vi "4461 - AI Read Data.vi"(8 "sampling info":cluster{"Fs":dbl, "#s":dbl}={"Fs"=1000.0, "#s"=1000.0} {"Fs" format="%.2p"}, 10 "AI Block Size":i32=5000, 11 "AI task":refnum<k21>[](array[refnum])=["", ""]) -> (1 "Backlog":u8(slide) scale=0.0..100.0, 2 "Input Signals":dbl[][](array[numeric]), 3 "Input Signals":waveform(dbl)[](array[waveform]))   [LabVIEW 2013]
uses:
  <vilib>/DAQmx/read.llb/DAQmx Read (Analog 2D DBL NChan NSamp).vi
  <resource>/objmgr/daqmx.rc
  <vilib>/DAQmx/read.llb/DAQmx Read (Analog 1D Wfm NChan NSamp).vi
panel:
  in  "AI Rate":dbl=10000.0 format="%.2f"
  in  "AI Buffer Size (s)":i32=10
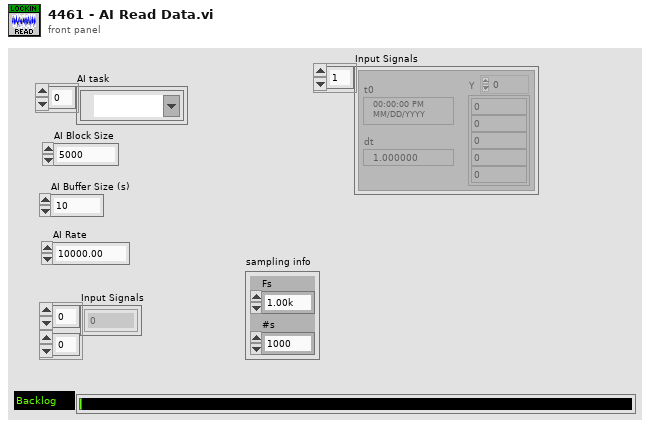
[diagram p1: front panel]
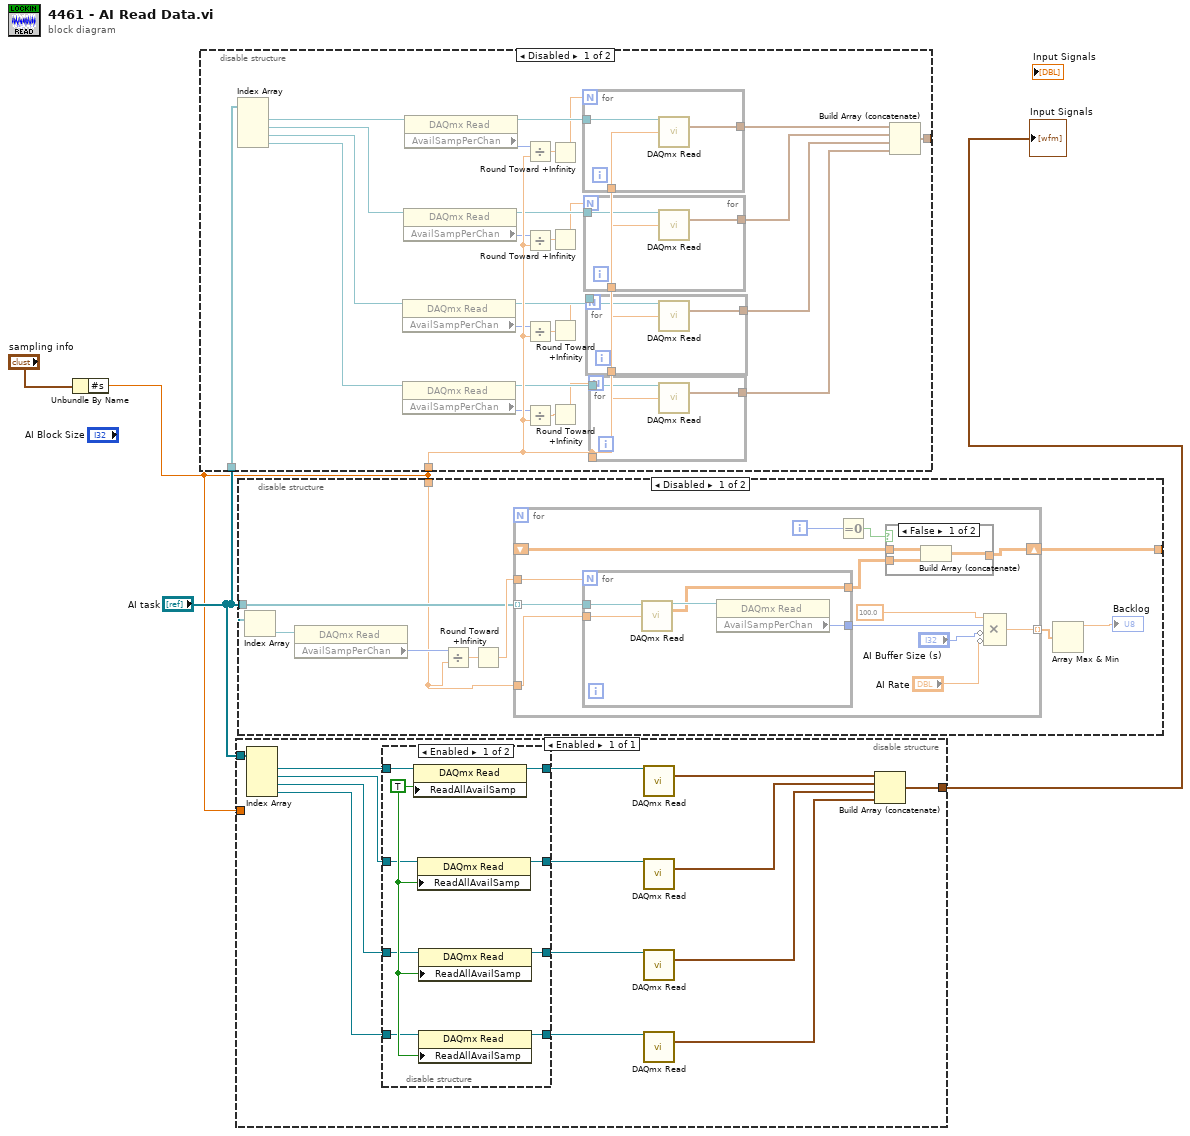
[diagram p0: block diagram]
diagram:
  n1 = Unbundle By Name("sampling info") -> ("#s"=w1:dbl)
  n2 = disable-structure shown="Disabled" {
    disable-tunnel: "AI task" -> [w31 _]
    disable-tunnel: w1 -> [w30 _]
    disable-tunnel: [w5 _] -> _
    frame Disabled {
      n3 = Index Array(array=w31) -> (element #1=w22:refnum<k21>, element #2=w23:refnum<k21>, element #3=w24:refnum<k21>, element #4=w25:refnum<k21>)  [unwired: 4 in]
      n4 = property class="DAQmx Read"(reference=w24) -> (reference out=w19:refnum<k21>, "AvailSampPerChan"=w15:u32)  [unwired: 1 in, 1 out]
      n5 = property class="DAQmx Read"(reference=w25) -> (reference out=w18:refnum<k21>, "AvailSampPerChan"=w16:u32)  [unwired: 1 in, 1 out]
      n6 = property class="DAQmx Read"(reference=w23) -> (reference out=w20:refnum<k21>, "AvailSampPerChan"=w14:u32)  [unwired: 1 in, 1 out]
      n7 = property class="DAQmx Read"(reference=w22) -> (reference out=w21:refnum<k21>, "AvailSampPerChan"=w17:u32)  [unwired: 1 in, 1 out]
      n8 = Divide(x=w17, y=w30) -> (x/y=w13:dbl)
      n9 = Divide(x=w14, y=w30) -> (x/y=w12:dbl)
      n10 = Divide(x=w15, y=w30) -> (x/y=w11:dbl)
      n11 = Divide(x=w16, y=w30) -> (x/y=w10:dbl)
      n12 = Round Toward +Infinity(x=w13) -> (ceil(x): smallest int >= x=w6:dbl)
      n13 = Round Toward +Infinity(x=w12) -> (ceil(x): smallest int >= x=w7:dbl)
      n14 = Round Toward +Infinity(x=w11) -> (ceil(x): smallest int >= x=w8:dbl)
      n15 = Round Toward +Infinity(x=w10) -> (ceil(x): smallest int >= x=w9:dbl)
      n16 = for {
        N: w6 -> [_]
        tunnel: [w43] -> w26
        tunnel: w21 -> [w42]
        tunnel: w30 -> [w41]
        n17 = call-poly <vilib>:"DAQmx Read.vi"("task/channels in"=w42, "number of samples per channel"=w41) -> ("data"=w43:waveform(dbl)[])  [unwired: 11 in, 2 out]
      }
      n18 = for {
        N: w7 -> [_]
        tunnel: [w40] -> w27
        tunnel: w20 -> [w39]
        tunnel: w30 -> [w38]
        n19 = call-poly <vilib>:"DAQmx Read.vi"("task/channels in"=w39, "number of samples per channel"=w38) -> ("data"=w40:waveform(dbl)[])  [unwired: 11 in, 2 out]
      }
      n20 = for {
        N: w8 -> [_]
        tunnel: [w37] -> w28
        tunnel: w19 -> [w36]
        tunnel: w30 -> [w35]
        n21 = call-poly <vilib>:"DAQmx Read.vi"("task/channels in"=w36, "number of samples per channel"=w35) -> ("data"=w37:waveform(dbl)[])  [unwired: 11 in, 2 out]
      }
      n22 = for {
        N: w9 -> [_]
        tunnel: [w34] -> w29
        tunnel: w18 -> [w33]
        tunnel: w30 -> [w32]
        n23 = call-poly <vilib>:"DAQmx Read.vi"("task/channels in"=w33, "number of samples per channel"=w32) -> ("data"=w34:waveform(dbl)[])  [unwired: 11 in, 2 out]
      }
      n24 = Build Array (concatenate)(w26, w27, w28, w29) -> (w5:waveform(dbl)[])
    }
    frame Enabled {
    }
  }
  n25 = disable-structure shown="Enabled" {
    disable-tunnel: "AI task" -> [w57]
    disable-tunnel: w1 -> [_]
    disable-tunnel: [w44] -> w4
    frame Enabled {
      n26 = Index Array(array=w57) -> (element #1=w56:refnum<k21>, element #2=w51:refnum<k21>, element #3=w50:refnum<k21>, element #4=w49:refnum<k21>)  [unwired: 4 in]
      n27 = disable-structure shown="Enabled" {
        disable-tunnel: w56 -> [w66 w70]
        disable-tunnel: [w65 w70] -> w55
        disable-tunnel: [w64 w67] -> w54
        disable-tunnel: [w63 w68] -> w53
        disable-tunnel: [w62 w69] -> w52
        disable-tunnel: w51 -> [w60 w69]
        disable-tunnel: w50 -> [w59 w68]
        disable-tunnel: w49 -> [w58 w67]
        frame Enabled {
          w61 = TRUE ("ReadAllAvailSamp")
          n28 = property class="DAQmx Read"(reference=w66, "ReadAllAvailSamp"=w61) -> (reference out=w65:refnum<k21>)  [unwired: 1 in, 1 out]
          n29 = property class="DAQmx Read"(reference=w60, "ReadAllAvailSamp"=w61) -> (reference out=w62:refnum<k21>)  [unwired: 1 in, 1 out]
          n30 = property class="DAQmx Read"(reference=w59, "ReadAllAvailSamp"=w61) -> (reference out=w63:refnum<k21>)  [unwired: 1 in, 1 out]
          n31 = property class="DAQmx Read"(reference=w58, "ReadAllAvailSamp"=w61) -> (reference out=w64:refnum<k21>)  [unwired: 1 in, 1 out]
        }
        frame Disabled {
        }
      }
      n32 = call-poly <vilib>:"DAQmx Read.vi"("task/channels in"=w55) -> ("data"=w48:waveform(dbl)[])  [unwired: 12 in, 2 out]
      n33 = call-poly <vilib>:"DAQmx Read.vi"("task/channels in"=w52) -> ("data"=w47:waveform(dbl)[])  [unwired: 12 in, 2 out]
      n34 = call-poly <vilib>:"DAQmx Read.vi"("task/channels in"=w53) -> ("data"=w46:waveform(dbl)[])  [unwired: 12 in, 2 out]
      n35 = call-poly <vilib>:"DAQmx Read.vi"("task/channels in"=w54) -> ("data"=w45:waveform(dbl)[])  [unwired: 12 in, 2 out]
      n36 = Build Array (concatenate)(w48, w47, w46, w45) -> (w44:waveform(dbl)[])
    }
  }
  "Input Signals" <- w4
  n37 = disable-structure shown="Disabled" {
    disable-tunnel: [w73 _] -> _
    disable-tunnel: "AI task" -> [w72 _]
    disable-tunnel: w1 -> [w71 _]
    frame Disabled {
      n38 = Index Array(array=w72) -> (element=w77:refnum<k21>)  [unwired: 1 in]
      n39 = property class="DAQmx Read"(reference=w77) -> ("AvailSampPerChan"=w76:u32)  [unwired: 1 in, 2 out]
      n40 = Divide(x=w76, y=w71) -> (x/y=w75:dbl)
      n41 = Round Toward +Infinity(x=w75) -> (ceil(x): smallest int >= x=w74:dbl)
      n42 = for {
        tunnel: w72 -> [w84] mode=indexing
        tunnel: [w90] -> w79 mode=indexing
        shift-right: [w85] -> w73
        shift-left: _ -> [w87]
        tunnel: w74 -> [w83]
        tunnel: w71 -> [w82]
        i -> [w88]
        n43 = for {
          N: w83 -> [_]
          tunnel: [w100] -> w86
          tunnel: [w99] -> w92
          tunnel: w84 -> [w98]
          tunnel: w82 -> [w97]
          n44 = call-poly <vilib>:"DAQmx Read.vi"("task/channels in"=w98, "number of samples per channel"=w97) -> ("task out"=w101:refnum<k21>, "data"=w100:dbl[][])  [unwired: 11 in, 1 out]
          n45 = property class="DAQmx Read"(reference=w101) -> ("AvailSampPerChan"=w99:u32)  [unwired: 1 in, 2 out]
        }
        n46 = Equal To 0?(x=w88) -> (x = 0?=w89:bool)
        n47 = case shown="False" w89 {
          tunnel: w87 -> [w93 _]
          tunnel: w86 -> [w95 w96]
          tunnel: [w94 w96] -> w85
          frame False {
            n48 = Build Array (concatenate)(w93, w95) -> (w94:dbl[][])
          }
          frame True {
          }
        }
        n49 = Compound Arithmetic op=MULTIPLY(100.0 ("value"), w92, invert "AI Buffer Size (s)", invert "AI Rate") -> (w90:dbl)
      }
      n50 = Array Max & Min(array=w79) -> (max value=→"Backlog":dbl)  [unwired: 3 out]
    }
    frame Enabled {
    }
  }
